vi "Exit Labiew.vi"(8 "错误输入（无错误）":errorcluster) -> (0 "错误输出":errorcluster)   [LabVIEW 2012, in "Application.lvlib"]
uses:
  Application.lvlib
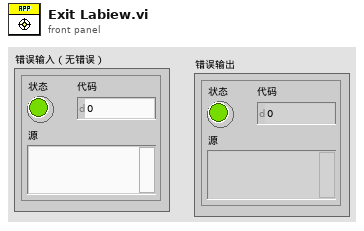
[diagram p1: front panel]
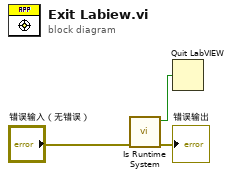
[diagram p0: block diagram]
diagram:
  n1 = call "Is Runtime System.vi"("错误输入（无错误）"="错误输入（无错误）") -> ("错误输出"=→"错误输出":errorcluster, "Is Runtime?"=w3:bool)  [unwired: 9 in]
  n2 = Quit LabVIEW(quit? (T)=w3) -> ()
